vi "VISA Query.vi"(8 "error in (no error)":errorcluster, 9 "Timeout (2000 ms)":i32=2000, 10 "Command":string, 11 "VISA resource name":refnum<visa-resource-name>) -> (0 "error out":errorcluster, 1 "Bytes Read":i32, 2 "Response":string, 3 "VISA resource name out":refnum<visa-resource-name>, 4 "Bytes Written":i32)   [LabVIEW 2019]
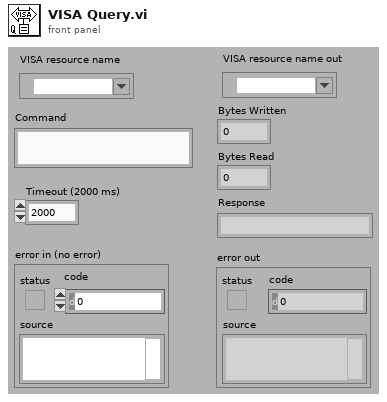
[diagram p1: front panel]
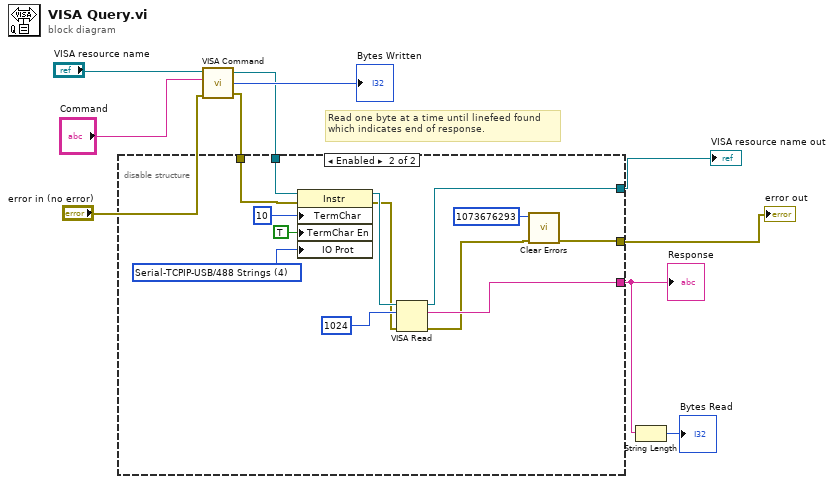
[diagram p0: block diagram]
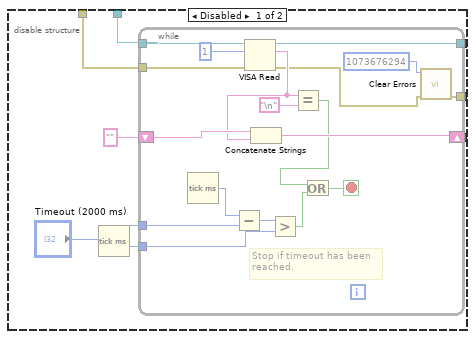
[diagram p2: hidden frame]
diagram:
  # "Read one byte at a time until linefeed found\nwhich indicates end of response."
  n1 = call "VISA Command.vi"("error in (no error)"="error in (no error)", "Command"="Command", "VISA resource name"="VISA resource name") -> ("error out"=w9:errorcluster, "bytes written"=→"Bytes Written":i32, "VISA resource name out"=w7:refnum<visa-resource-name>)  [unwired: 1 in]
  n2 = disable-structure shown="Enabled" {
    disable-tunnel: w9 -> [w18 w41]
    disable-tunnel: w7 -> [w17 w49]
    disable-tunnel: [w16 w45] -> w4
    disable-tunnel: [w15 w43] -> w3
    disable-tunnel: [w11 w38] -> w1
    frame Disabled {
      n3 = Tick Count (ms)() -> (millisecond timer value=w13:u32)
      n4 = while {
        tunnel: w17 -> [w24]
        tunnel: [w36] -> w16
        tunnel: w18 -> [w35]
        shift-right: [w31] -> w15
        shift-left: "" -> [w33]
        tunnel: "Timeout (2000 ms)" -> [w25]
        tunnel: w13 -> [w29]
        tunnel: [w20] -> w11
        stop <- w22 stop-if-true
        # "Stop if timeout has been\nreached."
        n5 = Tick Count (ms)() -> (millisecond timer value=w30:u32)
        n6 = Subtract(x=w30, y=w29) -> (x-y=w28:u32)
        n7 = VISA Read(VISA resource name=w24, byte count=u32 1 ("bytes to read"), error in (no error)=w35) -> (VISA resource name out=w36:refnum<visa-resource-name>, read buffer=w32:string, error out=w19:errorcluster)  [unwired: 1 out]
        n8 = Concatenate Strings(w33, w32) -> (w31:string)
        n9 = Greater?(x=w28, y=w25) -> (0:w27:bool)
        n10 = Equal?(x=w32, y="\n") -> (x = y?=w26:bool)
        n11 = Or(x=w26, y=w27) -> (x .or. y?=w22:bool)
        n12 = call <vilib>:"Clear Errors.vi"("error in (no error)"=w19, "specific error code to clear (0: all)"=1073676294) -> ("error out"=w20:errorcluster)  [unwired: 4 in, 1 out]
      }
    }
    frame Enabled {
      w47 = u16 4 items=["Normal"=1, "VXI/FDC"=2, "GPIB/HS488"=3, "Serial-TCPIP-USB/488 Strings"=4, "USBTMC/Vendor-Specific"=5] ("Message Based Settings:IO Protocol")
      n13 = property class="Instr"(reference=w49, error in=w41, "TermChar"=u8 10 ("Message Based Settings:Termination Character"), "TermChar En"=TRUE ("Message Based Settings:Termination Character Enable"), "IO Prot"=w47) -> (reference out=w46:refnum<visa-resource-name>, error out=w40:errorcluster)
      n14 = VISA Read(VISA resource name=w46, byte count=u32 1024, error in (no error)=w40) -> (VISA resource name out=w45:refnum<visa-resource-name>, read buffer=w43:string, error out=w39:errorcluster)  [unwired: 1 out]
      n15 = call <vilib>:"Clear Errors.vi"("error in (no error)"=w39, "specific error code to clear (0: all)"=1073676293) -> ("error out"=w38:errorcluster)  [unwired: 4 in, 1 out]
    }
  }
  "error out" <- w1
  "Response" <- w3
  "VISA resource name out" <- w4
  n16 = String Length(string=w3) -> (length=→"Bytes Read":i32)
